vi "PV OnTool Inert gas system.vi"(8 "error in (no error)":errorcluster, 9 "PV OnTool Inert gas - Cluster":T1 {"Parameter" items=[" Sealing gas valve", " Flushing gas valve", " Gas ballast valve         ", " Direct control output K1   ", " Operating mode innert gas system", " Purge gas system OK  (read only)"]}, 10 "Adress of unit":u16=1 max=999 step=1, 11 "VISA session":refnum<visa-resource-name>) -> (0 "error out":errorcluster, 2 "response (data)":string, 3 "dup VISA session":refnum<visa-resource-name>)   [LabVIEW 2021, in "Pfeiffer Vacuum.lvlib"]
doc: "There are 6 parameters available, only one of which can be enabled at a time. \n\n0 - Sealing gas valve (default) (Para.050)\n1 - Flushing gas valve (Para.051)\n2 - Gas ballast valve (Para.052)\n3 - Direct control output K1 (Para.053)\n4 - Operating mode inert gas system (Para.054)\n5 - Purge gas system OK (read only) (Para.344)\n\nNote: The 1 controls right of this one will set the appropriate values for the selected parameter. Any settings for an parameter that is not selected will be ignored. If a value is out of range, it will be changed to either the upper or the lower limit of the range."
uses:
  <instrlib>/Pfeiffer Vacuum/Pfeiffer Vacuum.lvlib
  <instrlib>/Pfeiffer Vacuum/Public/OnTool/PV OnTool Inert Gas System - Cluster.ctl
panel:
  # "Sealing gas valve                                       :\n Flushing gas valve                                     : \n Gas ballast valve                                        :\n Direct control output K1                           :\n Operating mode innert gas system        :"
  # "<--------------\n            off\n            off\n            off\n            off\n            automatic"
  # "----------->                \non  \non  \non  \non  \n              User control"
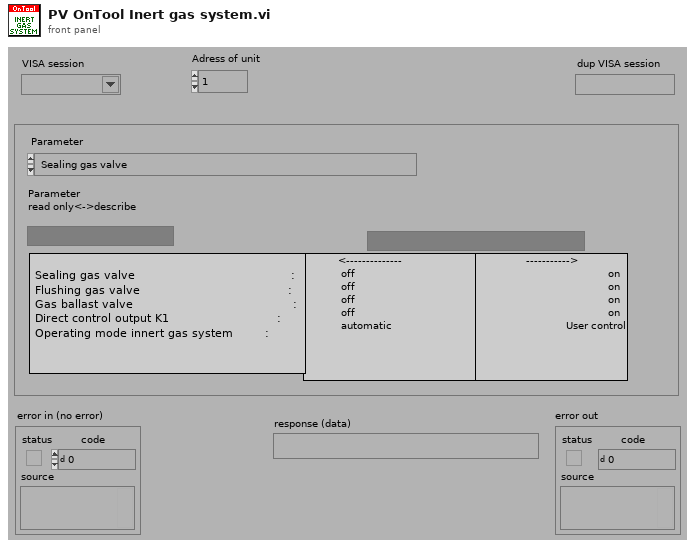
[diagram p1: front panel]
types:
  T1 = typedef "Pfeiffer Vacuum.lvlib/PV OnTool Inert Gas System - Cluster.ctl" = cluster{"Parameter":u16, "Parameter\nread only<->describe":bool, "off<->on":bool}
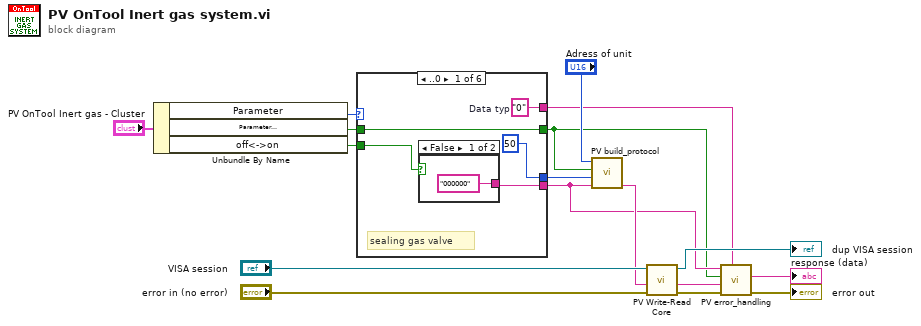
[diagram p0: block diagram]
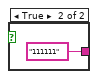
[diagram p2: hidden frame]
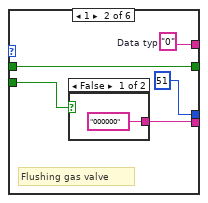
[diagram p3: hidden frame]
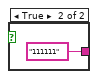
[diagram p4: hidden frame]
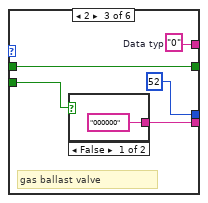
[diagram p5: hidden frame]
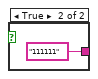
[diagram p6: hidden frame]
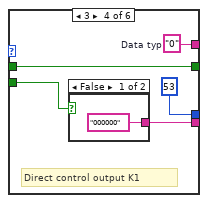
[diagram p7: hidden frame]
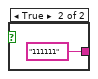
[diagram p8: hidden frame]
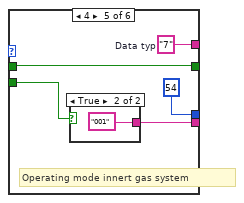
[diagram p9: hidden frame]
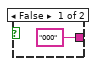
[diagram p10: hidden frame]
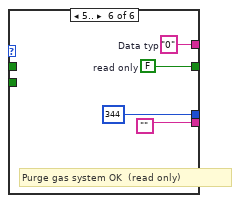
[diagram p11: hidden frame]
diagram:
  n1 = Unbundle By Name("PV OnTool Inert gas - Cluster") -> ("Parameter"=w14:u16, "Parameter\nread only<->describe"=w13:bool, "off<->on"=w12:bool)
  n2 = case shown="..0" w14 {
    tunnel: [u16 50 ("Parameter-number") u16 51 ("Parameter-number") u16 52 ("Parameter-number") u16 53 ("Parameter-number") u16 54 ("Parameter-number") u16 344 ("Parameter-number")] -> w16
    tunnel: [w20 w27 w34 w41 w47 ""] -> w4
    tunnel: [w21 w28 w36 w42 w49 w56] -> w3
    tunnel: w13 -> [w21 w28 w36 w42 w49 _]
    tunnel: w12 -> [w19 w26 w33 w40 w48 _]
    tunnel: [w18 w25 w32 w39 w46 w53] -> w5
    frame ..0 {
      w18 = "0"  # Data typ
      # "sealing gas valve"
      n3 = case shown="False" w19 {
        tunnel: ["000000" ("Data") "111111" ("Data")] -> w20
        frame False {
        }
        frame True {
        }
      }
    }
    frame 1 {
      w25 = "0"  # Data typ
      # "Flushing gas valve"
      n4 = case shown="False" w26 {
        tunnel: ["000000" ("Data") "111111" ("Data")] -> w27
        frame False {
        }
        frame True {
        }
      }
    }
    frame 2 {
      w32 = "0"  # Data typ
      # "gas ballast valve"
      n5 = case shown="False" w33 {
        tunnel: ["000000" ("Data") "111111" ("Data")] -> w34
        frame False {
        }
        frame True {
        }
      }
    }
    frame 3 {
      w39 = "0"  # Data typ
      # "Direct control output K1"
      n6 = case shown="False" w40 {
        tunnel: ["000000" ("Data") "111111" ("Data")] -> w41
        frame False {
        }
        frame True {
        }
      }
    }
    frame 4 {
      w46 = "7"  # Data typ
      # "Operating mode innert gas system"
      n7 = case shown="True" w48 {
        tunnel: ["000" ("Data") "001" ("Data")] -> w47
        frame False {
        }
        frame True {
        }
      }
    }
    frame 5.. {
      w53 = "0"  # Data typ
      w56 = FALSE  # read only
      # "Purge gas system OK  (read only)"
    }
  }
  n8 = call <instrlib>:"PV build_protocol.vi"("Data"=w4, "Parameter-number"=w16, "parameter\nread<->describe"=w3, "Adress"="Adress of unit") -> ("output"=w9:string)  [unwired: 3 in]
  n9 = call <instrlib>:"PV Write-Read Core.vi"("error in"="error in (no error)", "Write data in"=w9, "VISA session"="VISA session") -> ("error out"=w6:errorcluster, "response (data) out"=w7:string, "dup VISA session"=→"dup VISA session":refnum<visa-resource-name>)  [unwired: 2 in]
  n10 = call <instrlib>:"PV error_handling.vi"("Data Typ in"=w5, "error in"=w6, "response (data) in"=w7, "Parameter\nread only<->describe"=w3, "data in"=w4) -> ("error out"=→"error out":errorcluster, "Data out"=→"response (data)":string)  [unwired: 4 in, 1 out]
